vi "aquireIonGuage.vi"(10 "Sample Rate (1/s)":dbl, 11 "Number of Samples":i32) -> (1 "Voltage":dbl[](array[numeric]), 2 "Pressure":dbl[](array[numeric]), 3 "Time":dbl[](array[numeric]))   [LabVIEW 2011]
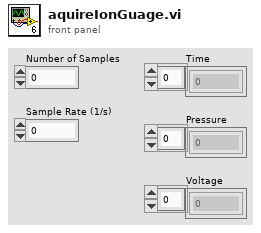
[diagram p1: front panel]
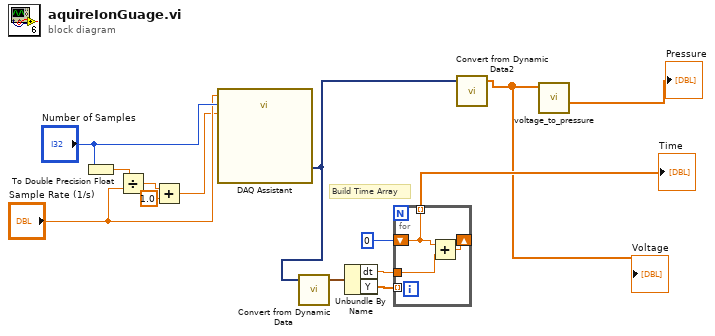
[diagram p0: block diagram]
diagram:
  # "Build Time Array"
  n1 = To Double Precision Float(number="Number of Samples") -> (double precision float=w5:dbl)
  n2 = Divide(x=w5, y="Sample Rate (1/s)") -> (x/y=w3:dbl)
  n3 = Add(x=w3, y=1.0) -> (x+y=w1:dbl)
  n4 = call "DAQ Assistant"("rate"="Sample Rate (1/s)", "number of samples"="Number of Samples", "timeout (s)"=w1) -> ("data"=w11:dynamicdata)  [unwired: 14 in, 2 out]
  n5 = call "Convert from Dynamic Data"("Dynamic Data Type"=w11) -> ("Waveform"=w9:waveform(dbl))  [unwired: 3 in]
  n6 = Unbundle By Name(w9) -> ("dt"=w8:dbl, "Y"=w7:dbl[])
  n7 = for {
    shift-right: [w16] -> _
    shift-left: 0 -> [w15]
    tunnel: w8 -> [w17]
    tunnel: [w15] -> w14 mode=indexing
    tunnel: w7 -> [_] mode=indexing
    n8 = Add(x=w15, y=w17) -> (x+y=w16:dbl)
  }
  "Time" <- w14
  n9 = call "Convert from Dynamic Data2"("Dynamic Data Type"=w11) -> ("Array"=w12:dbl[])  [unwired: 3 in]
  "Voltage" <- w12
  n10 = call "voltage_to_pressure.vi"("Voltage In"=w12) -> ("Pressure Out"=→"Pressure":dbl[])  [unwired: 8 in, 2 out]
